vi "GetFrontPanel.vi"(8 "ErrorIn":errorcluster, 11 "ObjectIn":refnum<class "YAFTAF.lvclass">) -> (0 "ErrorOut":errorcluster, 2 "FrontPanelControl":refnum<class "FrontPanelControl.lvclass">, 3 "ObjectOut":refnum<class "YAFTAF.lvclass">)   [LabVIEW 2021, in "YAFTAF.lvclass"]
doc: "Retrieve the FrontPanelControl for controlling the state of the user interface front panel"
uses:
  YAFTAF.lvclass
  Library_UserInterface_FrontPanelControl/FrontPanelControl/FrontPanelControl.lvclass
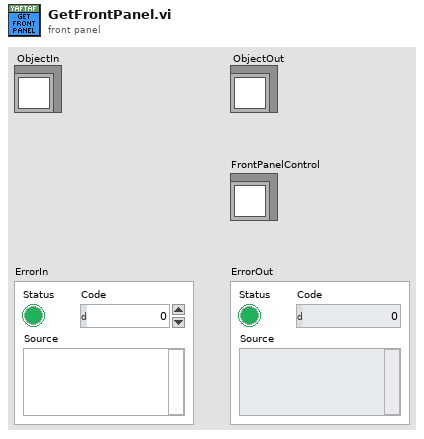
[diagram p1: front panel]
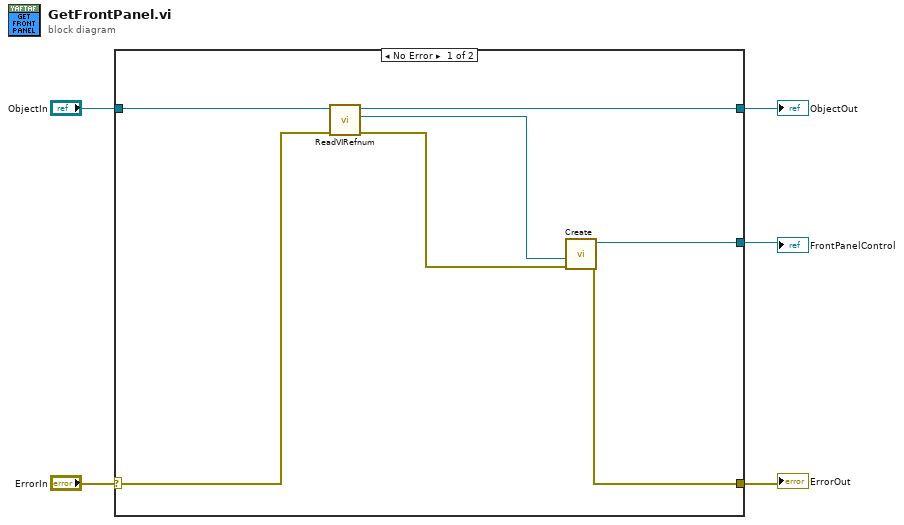
[diagram p0: block diagram]
diagram:
  n1 = case shown="No Error" "ErrorIn" {
    selector: "ErrorIn" -> [w12 w14]
    tunnel: [w10 w14] -> w4
    tunnel: [w9 w13] -> w2
    tunnel: "ObjectIn" -> [w8 w13]
    tunnel: [w6 _] -> w1
    frame No Error {
      n2 = call-dynamic "ReadVIRefnum.vi"("ErrorIn"=w12, "YActorIn"=w8) -> ("ErrorOut"=w11:errorcluster, "VIRefnum"=w7:refnum<vi>, "YActorOut"=w9:refnum<class "YAFTAF.lvclass">)  [unwired: 7 in]
      n3 = call "Create.vi"("ErrorIn"=w11, "VIRef"=w7) -> ("ErrorOut"=w10:errorcluster, "ObjectOut"=w6:refnum<class "FrontPanelControl.lvclass">)  [unwired: 8 in]
    }
    frame Error {
    }
  }
  "ErrorOut" <- w4
  "ObjectOut" <- w2
  "FrontPanelControl" <- w1
